vi "test2.vi"() -> ()   [LabVIEW 2019]
uses:
  <vilib>/Analysis/Matrix/Datatypes/RealMatrix.ctl
  <vilib>/Utility/file.llb/Write Delimited Spreadsheet (DBL).vi
  <vilib>/Analysis/Matrix/NI_Matrix.lvlib
panel:
  out "TimeOutCounter":i32
  out "ElapsedTime_M":dbl
  out "IMG_Contrast":dbl
  out "CurrentTrial":u32=1
  out "Jitter":dbl
  out "BaseITI":dbl
  out "VisStimDuration":dbl
  in  "Stop":bool
  out "Num trials":u32=204
  out "ISI Time":dbl
  out "Stim TS":dbl
  out "Output":dbl[][](array[numeric])
  out "Output frame":T1
  out "Array temp1":T1
  out "Elapsed Time":dbl
  out "Display":bool=TRUE
  out "Trial":u32=1
  out "reward":dbl[](array[numeric])
  out "stim_id":dbl[](array[numeric])
  out "stim_loaded":dbl
  out "Timings":dbl[](array[numeric])
  out "Stimuli Loaded?":bool
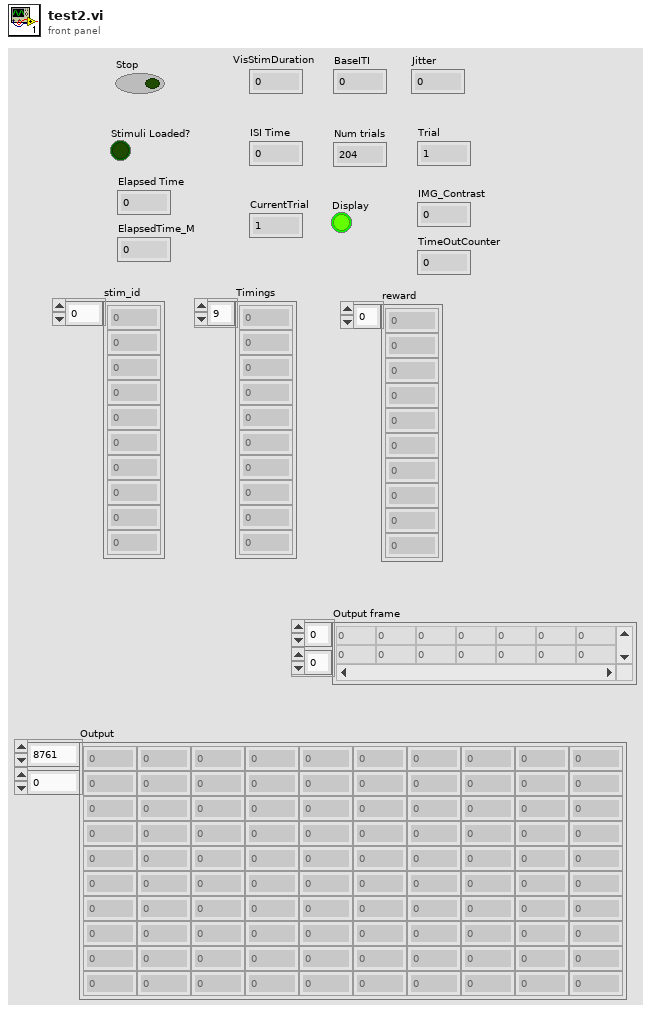
[diagram p1: front panel]
types:
  T1 = typedef "NI_Matrix.lvlib/RealMatrix.ctl" = dbl[][]
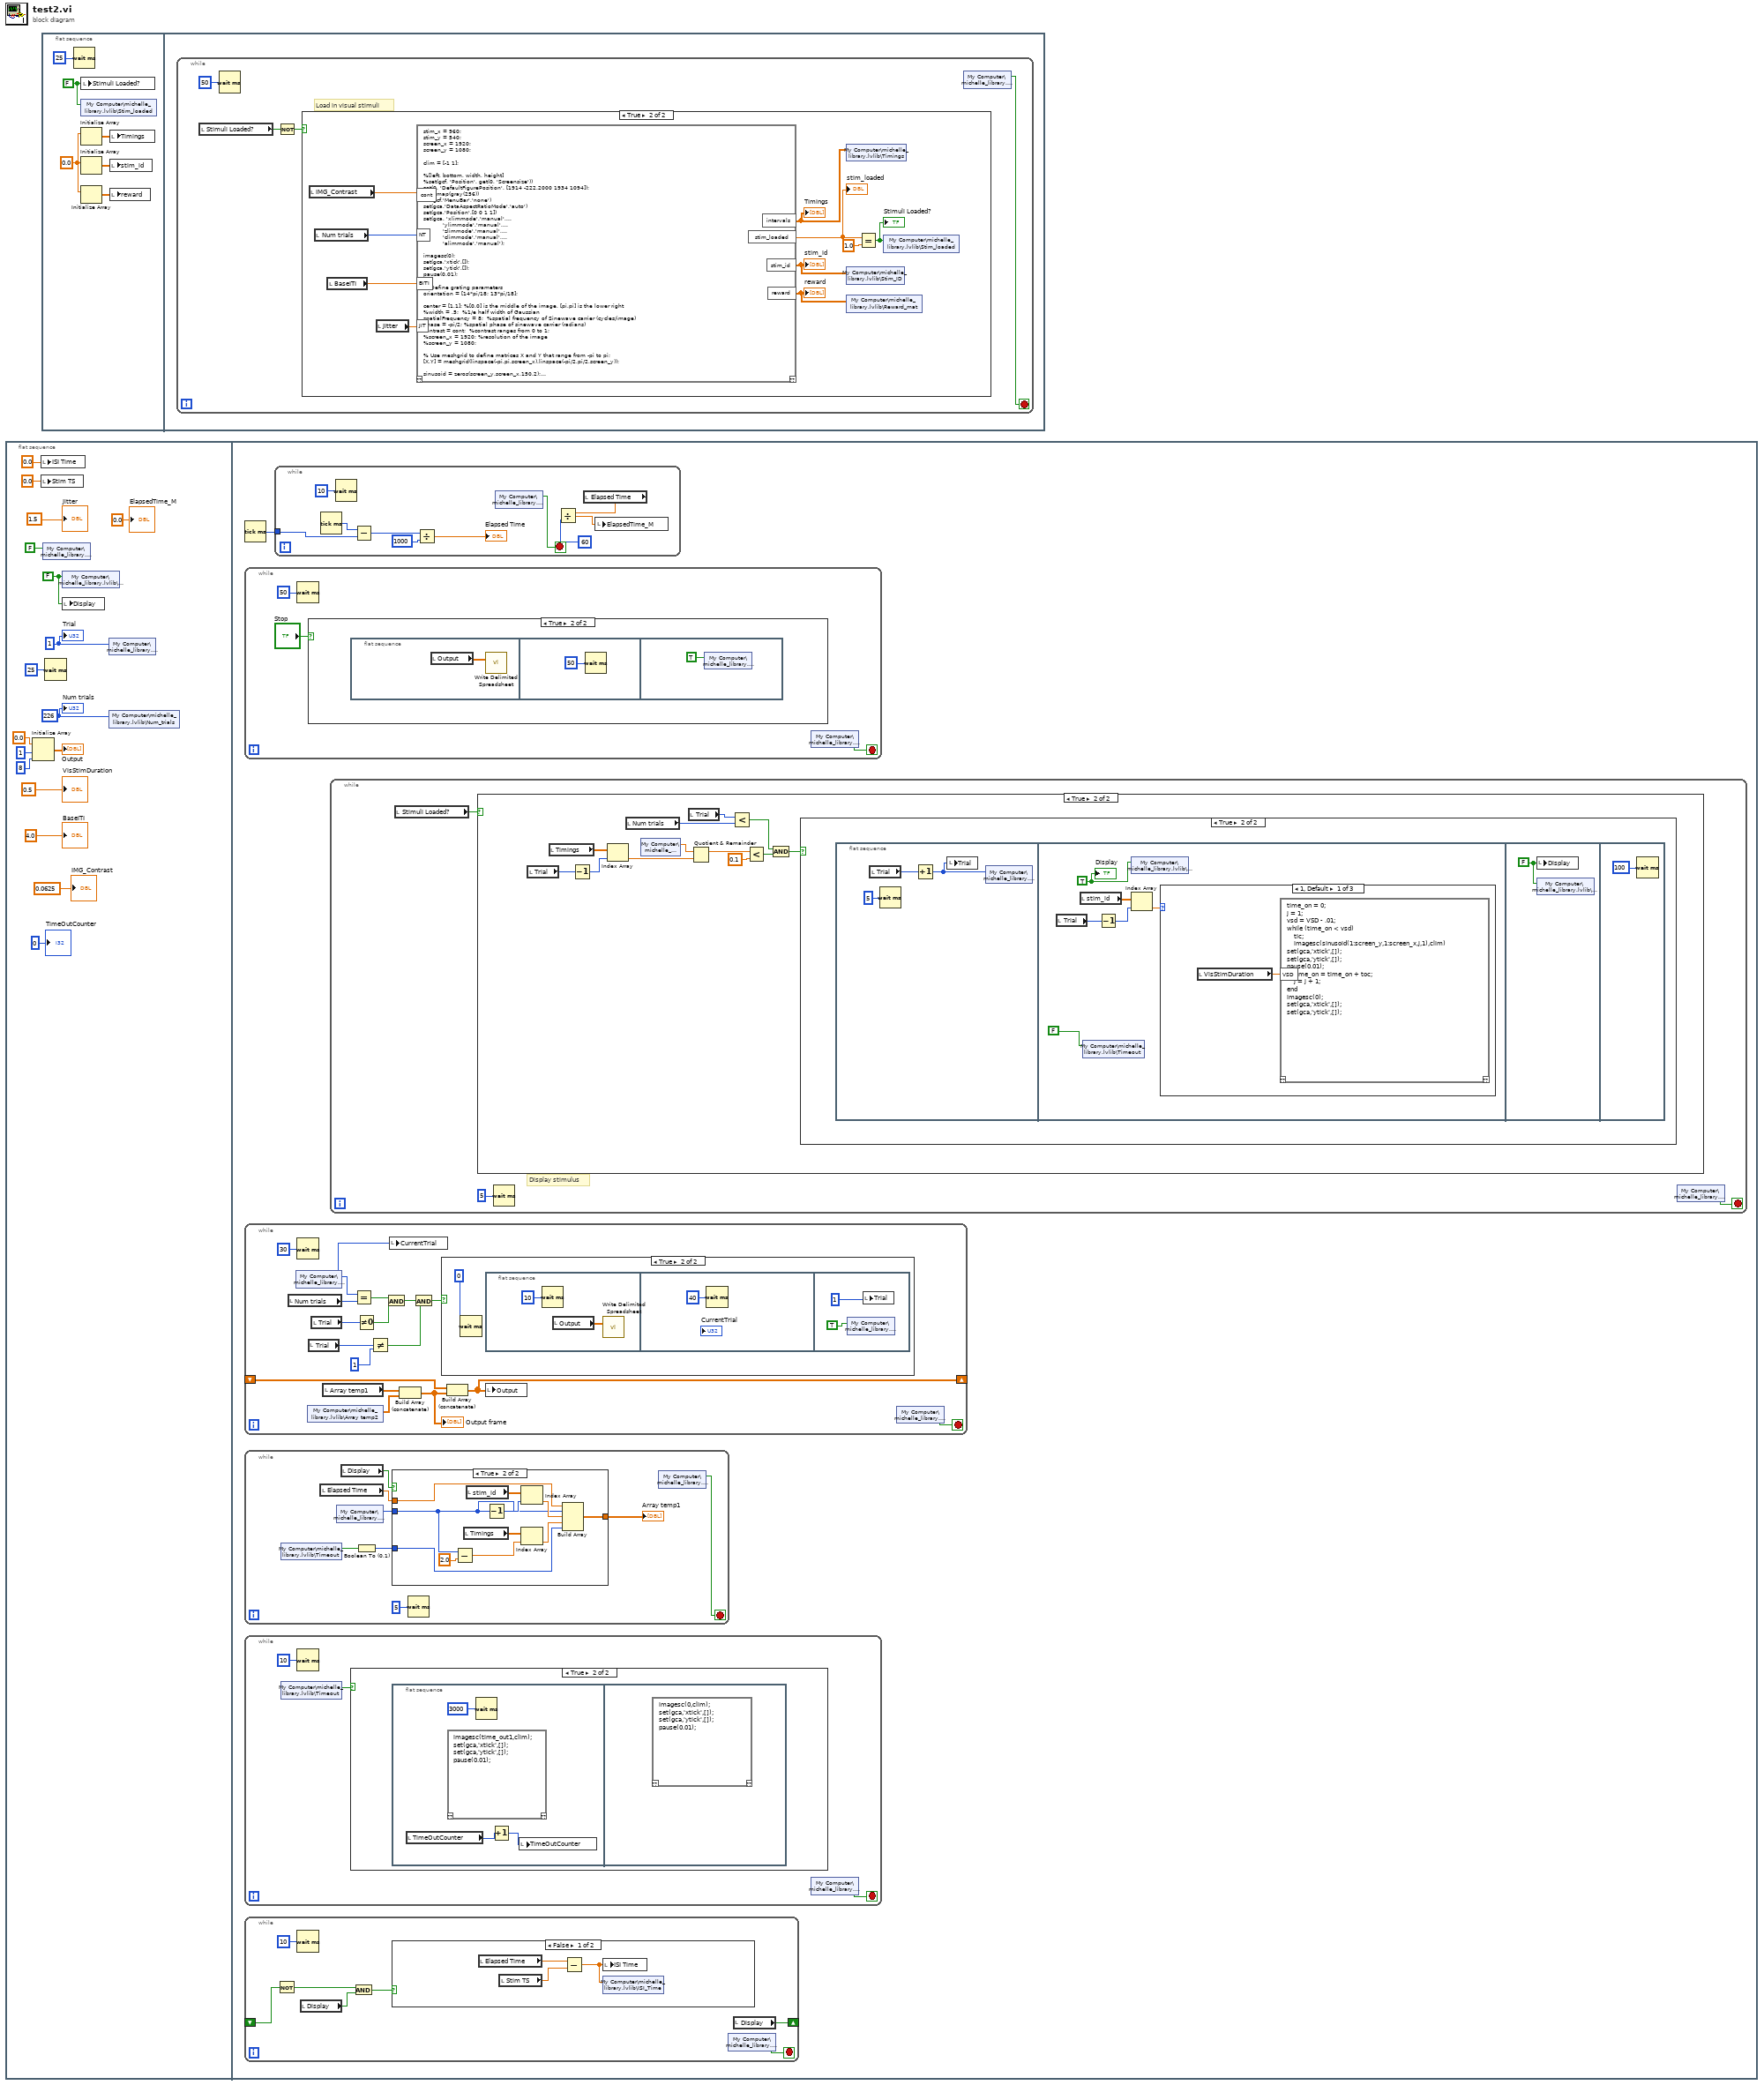
[diagram p0: block diagram]
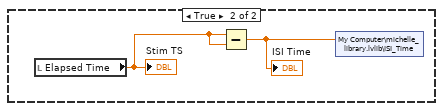
[diagram p5: hidden frame]
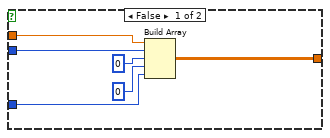
[diagram p6: hidden frame]
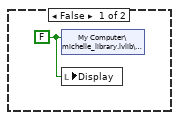
[diagram p9: hidden frame]
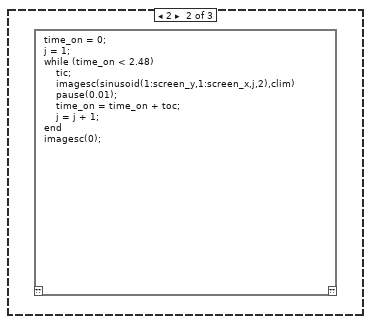
[diagram p10: hidden frame]
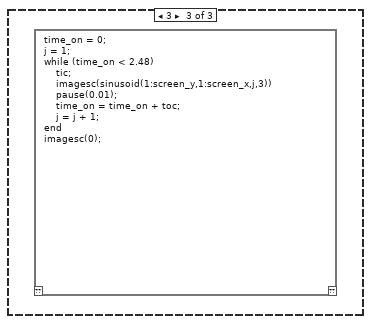
[diagram p11: hidden frame]
diagram:
  n1 = flat-sequence {
    frame #0 {
      w9 = u32 226
      w15 = FALSE ("Display")
      w17 = u32 1 ("Trial")
      n2 = Initialize Array(0.0 ("element"), 1 ("dimension size"), 8 ("dimension size")) -> (→"Output":dbl[][])
      n3 = local write "ISI Time"(0.0 ("ISI Time")) -> ()
      n4 = local write "Stim TS"(0.0 ("Stim TS")) -> ()
      n5 = shared-variable "My Computer\\michelle_library.lvlib\\Stop"(FALSE ("Stop")) -> ()  [unwired: 1 in, 1 out]
      n6 = Wait (ms)(milliseconds to wait=u32 25) -> ()  [unwired: 1 out]
      n7 = shared-variable "My Computer\\michelle_library.lvlib\\Display"(w15) -> ()  [unwired: 1 in, 1 out]
      n8 = local write "Display"(w15) -> ()
      n9 = shared-variable "My Computer\\michelle_library.lvlib\\Trial"(w17) -> ()  [unwired: 1 in, 1 out]
      n10 = shared-variable "My Computer\\michelle_library.lvlib\\Num_trials"(w9) -> ()  [unwired: 1 in, 1 out]
      "Trial" <- w17
      "Num trials" <- w9
      "VisStimDuration" <- 0.5
      "BaseITI" <- 4.0
      "Jitter" <- 1.5
      "IMG_Contrast" <- 0.0625
      "ElapsedTime_M" <- 0.0
      "TimeOutCounter" <- 0
    }
    frame #1 {
      n11 = Tick Count (ms)() -> (millisecond timer value=w18:u32)
      n12 = while {
        stop <- w21 stop-if-true
        n13 = Wait (ms)(milliseconds to wait=50) -> ()  [unwired: 1 out]
        n14 = case shown="True" "Stop" {
          frame False {
          }
          frame True {
            n15 = flat-sequence {
              frame #0 {
                n16 = local read "Output"() -> (w22:dbl[][])
                n17 = call-poly <vilib>:"Write Delimited Spreadsheet.vi"("2D data"=w22) -> ()  [unwired: 13 in, 2 out]
              }
              frame #1 {
                n18 = Wait (ms)(milliseconds to wait=50) -> ()  [unwired: 1 out]
              }
              frame #2 {
                n19 = shared-variable "My Computer\\michelle_library.lvlib\\Stop"(TRUE) -> ()  [unwired: 1 in, 1 out]
              }
            }
          }
        }
        n20 = shared-variable "My Computer\\michelle_library.lvlib\\Stop"() -> (w21:bool)  [unwired: 1 in, 1 out]
      }
      n21 = while {
        shift-right: [w91] -> _
        shift-left: _ -> [w92]
        stop <- w94 stop-if-true
        n22 = local read "Num trials"() -> (w87:u32)
        n23 = shared-variable "My Computer\\michelle_library.lvlib\\Trial"() -> (w78:u32)  [unwired: 1 in, 1 out]
        n24 = Wait (ms)(milliseconds to wait=u32 30) -> ()  [unwired: 1 out]
        n25 = shared-variable "My Computer\\michelle_library.lvlib\\Array temp2"() -> (w89:dbl[][])  [unwired: 1 in, 1 out]
        n26 = local read "Trial"() -> (w84:u32)
        n27 = local read "Trial"() -> (w85:u32)
        n28 = local read "Array temp1"() -> (w90:T1)
        n29 = Equal?(x=w78, y=w87) -> (x = y?=w86:bool)
        n30 = Not Equal To 0?(x=w85) -> (x != 0?=w81:bool)
        n31 = Not Equal?(x=w84, y=1) -> (x != y?=w83:bool)
        n32 = And(x=w86, y=w81) -> (x .and. y?=w79:bool)
        n33 = local write "CurrentTrial"(w78) -> ()
        n34 = Build Array (concatenate)(w90, w89) -> (w88:T1)
        "Output frame" <- w88
        n35 = And(x=w79, y=w83) -> (x .and. y?=w80:bool)
        n36 = case shown="True" w80 {
          frame False {
          }
          frame True {
            n37 = Wait (ms)(milliseconds to wait=0) -> ()  [unwired: 1 out]
            n38 = flat-sequence {
              frame #0 {
                n39 = Wait (ms)(milliseconds to wait=u32 10) -> ()  [unwired: 1 out]
                n40 = local read "Output"() -> (w97:dbl[][])
                n41 = call-poly <vilib>:"Write Delimited Spreadsheet.vi"("2D data"=w97) -> ()  [unwired: 13 in, 2 out]
              }
              frame #1 {
                n42 = Wait (ms)(milliseconds to wait=u32 40) -> ()  [unwired: 1 out]
              }
              frame #2 {
                n43 = shared-variable "My Computer\\michelle_library.lvlib\\Stop"(TRUE) -> ()  [unwired: 1 in, 1 out]
                n44 = local write "Trial"(1) -> ()
              }
            }
          }
        }
        n45 = Build Array (concatenate) ("Build Matrix")(w92, w88) -> (w91:T1)
        n46 = local write "Output"(w91) -> ()
        n47 = shared-variable "My Computer\\michelle_library.lvlib\\Stop"() -> (w94:bool)  [unwired: 1 in, 1 out]
      }
      n48 = while {
        stop <- w45 stop-if-true
        n49 = shared-variable "My Computer\\michelle_library.lvlib\\Timeout"() -> (w43:bool)  [unwired: 1 in, 1 out]
        n50 = local read "Elapsed Time"() -> (w49:dbl)
        n51 = shared-variable "My Computer\\michelle_library.lvlib\\Trial"() -> (w47:u32)  [unwired: 1 in, 1 out]
        n52 = local read "Display"() -> (w46:bool)
        n53 = Boolean To (0,1)(Boolean=w43) -> (0, 1=w44:i16)
        n54 = case shown="True" w46 {
          tunnel: w47 -> [w55 w58]
          tunnel: w49 -> [w56 w65]
          tunnel: [w54 w66] -> w48
          tunnel: w44 -> [w51 w60]
          frame False {
            n55 = Build Array(w56, w55, u32 0 ("milliseconds to wait"), 0, w51) -> (w54:T1)
          }
          frame True {
            n56 = Subtract(x=w58, y=2.0) -> (x-y=w57:dbl)
            n57 = local read "Timings"() -> (w63:dbl[])
            n58 = local read "stim_id"() -> (w67:dbl[])
            n59 = Decrement(x=w58) -> (x-1=w62:u32)
            n60 = Index Array(array=w67, index=w62) -> (element=w64:dbl)
            n61 = Index Array(array=w63, index=w57) -> (element=w61:dbl)
            n62 = Build Array(w65, w58, w64, w61, w60) -> (w66:T1)
          }
        }
        "Array temp1" <- w48
        n63 = Wait (ms)(milliseconds to wait=u32 5) -> ()  [unwired: 1 out]
        n64 = shared-variable "My Computer\\michelle_library.lvlib\\Stop"() -> (w45:bool)  [unwired: 1 in, 1 out]
      }
      n65 = while {
        stop <- w27 stop-if-true
        n66 = shared-variable "My Computer\\michelle_library.lvlib\\Timeout"() -> (w25:bool)  [unwired: 1 in, 1 out]
        n67 = Wait (ms)(milliseconds to wait=u32 10) -> ()  [unwired: 1 out]
        n68 = case shown="True" w25 {
          frame False {
          }
          frame True {
            n69 = flat-sequence {
              frame #0 {
                n70 = local read "TimeOutCounter"() -> (w29:i32)
                n71 = script code="imagesc(time_out1,clim);\nset(gca,'xtick',[]);\nset(gca,'ytick',[]);\npause(0.01);"() -> ()  [unwired: 1 in, 1 out]
                n72 = Wait (ms)(milliseconds to wait=u32 3000) -> ()  [unwired: 1 out]
                n73 = Increment(x=w29) -> (x+1=w28:i32)
                n74 = local write "TimeOutCounter"(w28) -> ()
              }
              frame #1 {
                n75 = script code="imagesc(0,clim);\nset(gca,'xtick',[]);\nset(gca,'ytick',[]);\npause(0.01);"() -> ()  [unwired: 1 in, 1 out]
              }
            }
          }
        }
        n76 = shared-variable "My Computer\\michelle_library.lvlib\\Stop"() -> (w27:bool)  [unwired: 1 in, 1 out]
      }
      n77 = while {
        shift-right: [w35] -> _
        shift-left: _ -> [w34]
        stop <- w37 stop-if-true
        n78 = Not(x=w34) -> (.not. x?=w33:bool)
        n79 = Wait (ms)(milliseconds to wait=u32 10) -> ()  [unwired: 1 out]
        n80 = local read "Display"() -> (w32:bool)
        n81 = And(x=w33, y=w32) -> (x .and. y?=w31:bool)
        n82 = case shown="False" w31 {
          frame False {
            n83 = local read "Elapsed Time"() -> (w38:dbl)
            n84 = local read "Stim TS"() -> (w40:dbl)
            n85 = Subtract(x=w38, y=w40) -> (x-y=w39:dbl)
            n86 = local write "ISI Time"(w39) -> ()
            n87 = shared-variable "My Computer\\michelle_library.lvlib\\ISI_Time"(w39) -> ()  [unwired: 1 in, 1 out]
          }
          frame True {
            n88 = local read "Elapsed Time"() -> (w41:dbl)
            "Stim TS" <- w41
            n89 = Subtract(x=w41, y=w41) -> (x-y=w42:dbl)
            "ISI Time" <- w42
            n90 = shared-variable "My Computer\\michelle_library.lvlib\\ISI_Time"(w42) -> ()  [unwired: 1 in, 1 out]
          }
        }
        n91 = shared-variable "My Computer\\michelle_library.lvlib\\Stop"() -> (w37:bool)  [unwired: 1 in, 1 out]
        n92 = local read "Display"() -> (w35:bool)
      }
      n93 = while {
        tunnel: w18 -> [w74]
        stop <- w71 stop-if-true
        n94 = Tick Count (ms)() -> (millisecond timer value=w75:u32)
        n95 = Wait (ms)(milliseconds to wait=u32 10) -> ()  [unwired: 1 out]
        n96 = Subtract(x=w75, y=w74) -> (x-y=w72:u32)
        n97 = Divide(x=w72, y=u32 1000) -> (x/y=→"Elapsed Time":dbl)
        n98 = shared-variable "My Computer\\michelle_library.lvlib\\Stop"() -> (w71:bool)  [unwired: 1 in, 1 out]
        n99 = local read "Elapsed Time"() -> (w68:dbl)
        n100 = Divide(x=w68, y=60) -> (x/y=w70:dbl)
        n101 = local write "ElapsedTime_M"(w70) -> ()
      }
      n102 = while {
        stop <- w102 stop-if-true
        # "Display stimulus"
        n103 = local read "Stimuli Loaded?"() -> (w101:bool)
        n104 = case shown="True" w101 {
          frame False {
          }
          frame True {
            n105 = local read "Trial"() -> (w104:u32)
            n106 = local read "Timings"() -> (w113:dbl[])
            n107 = Decrement(x=w104) -> (x-1=w105:u32)
            n108 = Index Array(array=w113, index=w105) -> (element=w112:dbl)
            n109 = local read "Num trials"() -> (w108:u32)
            n110 = shared-variable "My Computer\\michelle_library.lvlib\\ISI"() -> (w107:dbl)  [unwired: 1 in, 1 out]
            n111 = local read "Trial"() -> (w111:u32)
            n112 = Quotient & Remainder(x=w107, y=w112) -> (x-y*floor(x/y)=w115:dbl)  [unwired: 1 out]
            n113 = Less?(x=w111, y=w108) -> (x < y?=w110:bool)
            n114 = Less?(x=w115, y=0.1) -> (x < y?=w109:bool)
            n115 = And(x=w110, y=w109) -> (x .and. y?=w106:bool)
            n116 = case shown="True" w106 {
              frame False {
                w116 = FALSE ("Display")
                n117 = shared-variable "My Computer\\michelle_library.lvlib\\Display"(w116) -> ()  [unwired: 1 in, 1 out]
                n118 = local write "Display"(w116) -> ()
              }
              frame True {
                n119 = flat-sequence {
                  frame #0 {
                    n120 = local read "Trial"() -> (w119:u32)
                    n121 = Wait (ms)(milliseconds to wait=u32 5) -> ()  [unwired: 1 out]
                    n122 = Increment(x=w119) -> (x+1=w118:u32)
                    n123 = local write "Trial"(w118) -> ()
                    n124 = shared-variable "My Computer\\michelle_library.lvlib\\Trial"(w118) -> ()  [unwired: 1 in, 1 out]
                  }
                  frame #1 {
                    w124 = TRUE ("Boolean")
                    n125 = local read "Trial"() -> (w122:u32)
                    n126 = local read "stim_id"() -> (w125:dbl[])
                    n127 = shared-variable "My Computer\\michelle_library.lvlib\\Timeout"(FALSE) -> ()  [unwired: 1 in, 1 out]
                    n128 = Decrement(x=w122) -> (x-1=w121:u32)
                    n129 = shared-variable "My Computer\\michelle_library.lvlib\\Display"(w124) -> ()  [unwired: 1 in, 1 out]
                    n130 = Index Array(array=w125, index=w121) -> (element=w123:dbl)
                    n131 = case shown="1, Default" w123 {
                      frame 1, Default {
                        n132 = local read "VisStimDuration"() -> (w126:dbl)
                        n133 = script code="time_on = 0;\nj = 1;\nvsd = VSD - .01;\nwhile (time_on < vsd)\n    tic;\n    imagesc(sinusoid(1:screen_y,1:screen_x,j,1),clim)\nset(gca,'xtick',[]);\nset(gca,'ytick',[]);    \npause(0.01);\n    time_on = time_on + toc;\n    j = j + 1;\nend\nimagesc(0);\nset(gca,'xtick',[]);\nset(gca,'ytick',[]);"("VSD"=w126) -> ()  [unwired: 1 in, 1 out]
                      }
                      frame 2 {
                        n134 = script code="time_on = 0;\nj = 1;\nwhile (time_on < 2.48)\n    tic;\n    imagesc(sinusoid(1:screen_y,1:screen_x,j,2),clim)\n    pause(0.01);\n    time_on = time_on + toc;\n    j = j + 1;\nend\nimagesc(0);"() -> ()  [unwired: 1 in, 1 out]
                      }
                      frame 3 {
                        n135 = script code="time_on = 0;\nj = 1;\nwhile (time_on < 2.48)\n    tic;\n    imagesc(sinusoid(1:screen_y,1:screen_x,j,3))\n    pause(0.01);\n    time_on = time_on + toc;\n    j = j + 1;\nend\nimagesc(0);"() -> ()  [unwired: 1 in, 1 out]
                      }
                    }
                    "Display" <- w124
                  }
                  frame #2 {
                    w127 = FALSE ("Display")
                    n136 = local write "Display"(w127) -> ()
                    n137 = shared-variable "My Computer\\michelle_library.lvlib\\Display"(w127) -> ()  [unwired: 1 in, 1 out]
                  }
                  frame #3 {
                    n138 = Wait (ms)(milliseconds to wait=u32 100) -> ()  [unwired: 1 out]
                  }
                }
              }
            }
          }
        }
        n139 = Wait (ms)(milliseconds to wait=u32 5) -> ()  [unwired: 1 out]
        n140 = shared-variable "My Computer\\michelle_library.lvlib\\Stop"() -> (w102:bool)  [unwired: 1 in, 1 out]
      }
    }
  }
  n141 = flat-sequence {
    frame #0 {
      w131 = 0.0 ("element")
      w129 = FALSE ("Stimuli Loaded?")
      n142 = Wait (ms)(milliseconds to wait=u32 25) -> ()  [unwired: 1 out]
      n143 = local write "Stimuli Loaded?"(w129) -> ()
      n144 = shared-variable "My Computer\\michelle_library.lvlib\\Stim_loaded"(w129) -> ()  [unwired: 1 in, 1 out]
      n145 = Initialize Array(w131) -> (w133:dbl[])  [unwired: 1 in]
      n146 = Initialize Array(w131) -> (w132:dbl[])  [unwired: 1 in]
      n147 = Initialize Array(w131) -> (w130:dbl[])  [unwired: 1 in]
      n148 = local write "Timings"(w133) -> ()
      n149 = local write "stim_id"(w132) -> ()
      n150 = local write "reward"(w130) -> ()
    }
    frame #1 {
      n151 = while {
        stop <- w137 stop-if-true
        # "Load in visual stimuli"
        n152 = local read "Stimuli Loaded?"() -> (w136:bool)
        n153 = Wait (ms)(milliseconds to wait=u32 50) -> ()  [unwired: 1 out]
        n154 = Not(x=w136) -> (.not. x?=w135:bool)
        n155 = case shown="True" w135 {
          frame False {
          }
          frame True {
            n156 = local read "IMG_Contrast"() -> (w139:dbl)
            n157 = local read "Num trials"() -> (w142:u32)
            n158 = local read "BaseITI"() -> (w141:dbl)
            n159 = local read "Jitter"() -> (w140:dbl)
            n160 = script code="stim_x = 960;\nstim_y = 540;\nscreen_x = 1920;\nscreen_y = 1080;\n\nclim = [-1 1];\n\n%[left, bottom, width, height]\n%set(gcf, 'Position', get(0, 'Screensize'))\nset(0, 'DefaultFigurePosition', [1914 -222.2000 1934 1094]);\ncolormap(gray(256))\nset(gcf,'MenuBar','none')\nset(gca,'DataAspectRatioMode','auto')\nset(gca,'Position',[0 0 1 1])\nset(gca, 'xlimmode','manual',...\n           'ylimmode','manual',...\n           'zlimmode','manual',...\n           'climmode','manual',...\n           'alimmode','manual');\n\nimagesc(0);\nset(gca,'xtick',[]);\nset(gca,'ytick',[]);\npause(0.01);\n\n% Define grating parameters\norientation = [14*pi/18; 13*pi/18];\n\ncenter = [1,1]; %[0,0] is the middle of the image, [pi,pi] is the lower right\n%width = .5;  %1/e half width of Gaussian\nspatialFrequency = 8;  %spatial frequency of Sinewave carrier (cycles/image)\nphase = -pi/2; %spatial phase of sinewave carrier (radians)\ncontrast = cont;  %contrast ranges from 0 to 1;\n%screen_x = 1920; %resolution of the image  \n%screen_y = 1080;\n\n% Use meshgrid to define matrices X and Y that range from -pi to pi;\n[X,Y] = meshgrid(linspace(-pi,pi,screen_x),linspace(-pi/2,pi/2,screen_y));\n\nsinusoid = zeros(screen_y,screen_x,150,2);\ntime_out1 = ones(screen_y,screen_x)*-1;\ntime_out2 = zeros(screen_y,screen_x);\n%time_out(1,1) = 1;\n% Set up individual 4-d matrices (x, y, time, orientation) for movies of the drifting gratings at each\n% orientation\nfor j = 1:length(orientation)                                                            % Phase increase number here\n    ramp(1:screen_y,1:screen_x,j) = cos(orientation(j))*(X-center(1)) + sin(orientation(j))*(Y-center(2));     %  |\n    for i = 1:150 %Sets the number of frames to define gratings for                   V\n       sinusoid(1:screen_y,1:screen_x,i,j) = contrast*sin(spatialFrequency*ramp(1:screen_y,1:screen_x,j)-...\n           (phase+(2*pi*(i-1)*(-30)/360))); %Number before '/360' sets the phase increase\n    end\nend\n\n%intervals = [ones(1,41)*10 ones(1,41)*11 ones(1,41)*12 ones(1,41)*13 ones(1,40)*14];\njit = JIT;\njitter = rand(1,NT);\njitter = 2*jit*(jitter- .5);\nITIbase = BITI;\nintervals = [ones(1,NT)*ITIbase];\nintervals = intervals + jitter;\nstim_id = [ones(1,NT)*1];\n%reward = [ones(1,87)*1 ones(1,15)*0 ones(1,87)*1 ones(1,15)*0];\nreward = [ones(1,NT)*1];\n\nrand_idx1 = randperm(NT);\nrand_idx2 = randperm(NT);\nintervals = intervals(rand_idx2);\nstim_id = stim_id(rand_idx2);\nreward = reward(rand_idx2);\n\nstim_loaded = 1;" ("Script Node")("NT"=w142, "BITI"=w141, "JIT"=w140, "cont"=w139) -> ("stim_loaded"=w148:dbl, "intervals"=w143:dbl[], "stim_id"=w144:dbl[], "reward"=w146:dbl[])  [unwired: 1 in, 1 out]
            "stim_loaded" <- w148
            "Timings" <- w143
            "stim_id" <- w144
            "reward" <- w146
            n161 = shared-variable "My Computer\\michelle_library.lvlib\\Timings"(w143) -> ()  [unwired: 1 in, 1 out]
            n162 = shared-variable "My Computer\\michelle_library.lvlib\\Stim_ID"(w144) -> ()  [unwired: 1 in, 1 out]
            n163 = shared-variable "My Computer\\michelle_library.lvlib\\Reward_mat"(w146) -> ()  [unwired: 1 in, 1 out]
            n164 = Equal?(x=w148, y=1.0) -> (x = y?=w145:bool)
            "Stimuli Loaded?" <- w145
            n165 = shared-variable "My Computer\\michelle_library.lvlib\\Stim_loaded"(w145) -> ()  [unwired: 1 in, 1 out]
          }
        }
        n166 = shared-variable "My Computer\\michelle_library.lvlib\\Stop"() -> (w137:bool)  [unwired: 1 in, 1 out]
      }
    }
  }
